vi "Chronos TDMS Viewer Generate Graph and Labels.vi"(8 "error in (no error)":errorcluster, 11 "Limit Plot Map":T2) -> (0 "error out":errorcluster, 3 "Plot Settings":T1)   [LabVIEW 2021]
uses:
  GUI/Chronos cluster Map Limit Plots.ctl
  typedefs/Chronos cluster Plot Data and Limits.ctl
  cluster CC Channel from TDMS.ctl
  Chronos cluster Plot Settings.ctl
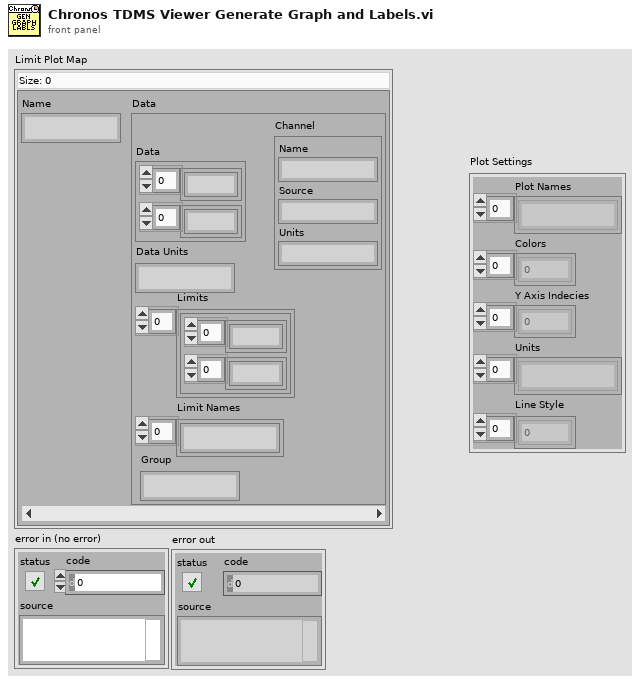
[diagram p1: front panel]
types:
  T1 = typedef "Chronos cluster Plot Settings.ctl" = cluster{"Plot Names":string[], "Colors":u32[], "Y Axis Indecies":i32[], "Units":string[], "Line Style":u8[]}
  T2 = typedef "Chronos cluster Map Limit Plots.ctl" = map{string, T3}
  T3 = typedef "Chronos cluster Plot Data and Limits.ctl" = cluster{"Data":cluster{dbl[], dbl[]}, "Data Units":string, "Limits":cluster{dbl[], dbl[]}[], "Limit Names":string[], "Channel":T4, "Group":string}
  T4 = typedef "cluster CC Channel from TDMS.ctl" = cluster{"Name":string, "Source":string, "Units":string}
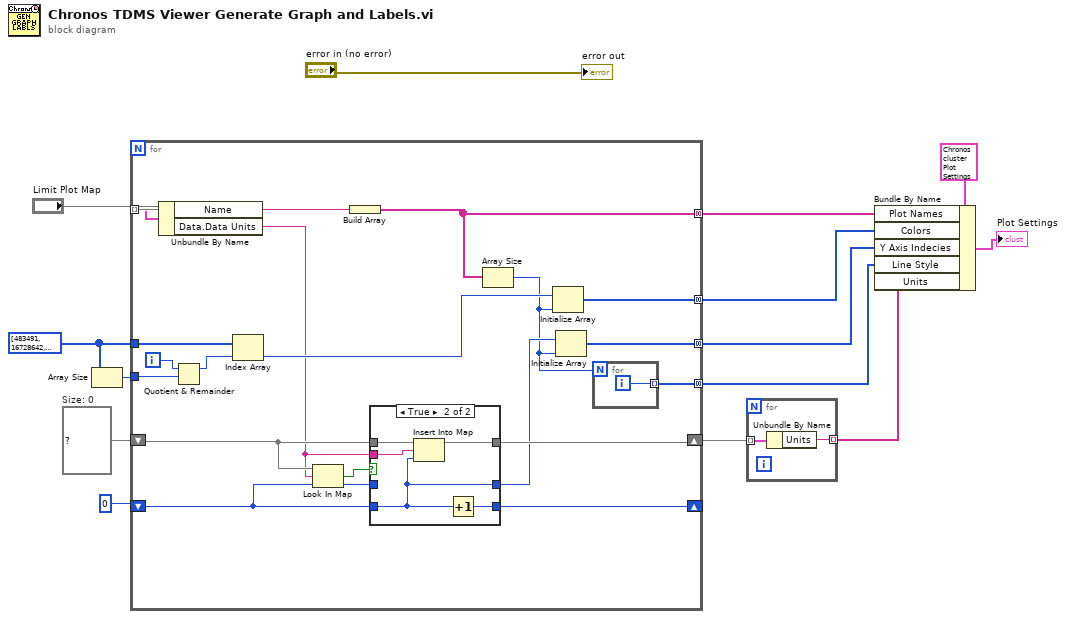
[diagram p0: block diagram]
diagram:
  w10 = map{string, i32} {}  # Size: 0
  w12 = u32[] [483491, 16728642, 982784, 4375295, 13827953, 13457919, 16757522, 4343295, 16728758, 5898228, 16777215, 16728642, 982784, 4375295, 13827953, 13457919, 16757522, 4343295] ("Colors")
  n1 = Array Size(array=w12) -> (size(s)=w11:i32)
  n2 = for {
    tunnel: [w20] -> w6 mode=concatenating
    tunnel: "Limit Plot Map" -> [w34] mode=indexing
    tunnel: [w32] -> w4 mode=concatenating
    tunnel: w12 -> [w31]
    tunnel: w11 -> [w28]
    shift-right: [w23] -> w8
    shift-left: w10 -> [w25]
    shift-right: [w22] -> _
    shift-left: 0 -> [w24]
    tunnel: [w18] -> w5 mode=concatenating
    tunnel: [w16] -> w2 mode=concatenating
    i -> [w29]
    n3 = Unbundle By Name(w34) -> ("Name"=w33:string, "Data.Data Units"=w15:string)
    n4 = Quotient & Remainder(x=w29, y=w28) -> (x-y*floor(x/y)=w30:i32)  [unwired: 1 out]
    n5 = Index Array(array=w31, index=w30) -> (element=w19:u32)
    n6 = Look In Map(map=w25, key=w15, default value=w24) -> (key not found?=w27:bool, value=w26:i32)
    n7 = Build Array(w33) -> (w20:string[])
    n8 = case shown="True" w27 {
      tunnel: w25 -> [w38 w43]
      tunnel: w15 -> [_ w42]
      tunnel: w24 -> [w37 w39]
      tunnel: [w37 w41] -> w22
      tunnel: [w38 w40] -> w23
      tunnel: w26 -> [w36 _]
      tunnel: [w36 w39] -> w21
      frame False {
      }
      frame True {
        n9 = Insert Into Map(map in=w43, key=w42, value=w39) -> (map out=w40:map{string, i32})  [unwired: 2 out]
        n10 = Increment(x=w39) -> (x+1=w41:i32)
      }
    }
    n11 = Array Size(array=w20) -> (size(s)=w17:i32)
    n12 = Initialize Array(w19, w17) -> (w18:u32[])
    n13 = Initialize Array(w21, w17) -> (w32:i32[])
    n14 = for {
      N: w17 -> [_]
      tunnel: [w35] -> w16 mode=indexing
      i -> [w35]
    }
  }
  n15 = for {
    tunnel: w8 -> [w45] mode=indexing
    tunnel: [w44] -> w1 mode=indexing
    n16 = Unbundle By Name(w45) -> ("Units"=w44:string)
  }
  n17 = Bundle By Name(cluster=T1 {"Plot Names"=["Channel 1", " Red Low", " Red Hi", " Yellow Low", " Yellow Hi"], "Colors"=[], "Y Axis Indecies"=[0, 0, 0, 0, 0], "Units"=["V"], "Line Style"=[]} ("Plot Settings"), "Plot Names"=w6, "Colors"=w5, "Y Axis Indecies"=w4, "Line Style"=w2, "Units"=w1) -> (→"Plot Settings":T1)
  "error out" <- "error in (no error)"
